vi "Insert Time Trace.vi"(4 "Anlaysis Info Cluster":T1={"Colour"=0, "Inst type"=enum."Pitot-static tube", "Inst name"="Manometer voltage", "Symbol"="U", "Code name"="", "Extra Info"="U", "Inst Array"=enum."PWA", "U"=0.0, "u^2"=0.0, "u^3"=0.0, "u^4"=0.0, "Skew_u"=0.0, "Kurt_u"=0.0, "Sd Error in Mean"=0.0, "% u'/U"=0.0, "X"=0.0, "Y"=0.0, "Z"=0.0, "Timescale integral Estimate"=0.0, "Sd Error in Variance"=0.0, "Calib File"=path "", "Calib Constants"=[], "Output Position"=FALSE, "Stats"=enum."None", "Av Sampling Rate"=0.0, "Av No of Samples"=0.0, "Total Meas Time (s)"=0.0, "OrigChName"="", "Max value"=0.0, "Min value"=0.0, "Req Sample Rate Hz"=0.0, "Sync Delay Time (s)"=0.0, "Ch No"=0, "Device"="", "Use Latest Calib"=FALSE, "Port"="", "Metadata Ch Names"=[], "Metadata Ch Values"=[], "Label"="", "chState"=enum."Solo", "Point Drift"=0.0, "inputConfig"=""} {"Kurt_u" format="%_3g"; "u^4" format="%_3g"; "u^3" format="%_3g"; "Sd Error in Variance" format="%_3g"; "u^2" format="%_3g"; "Sd Error in Mean" format="%_3g"; "U" format="%_3g"; "Sync Delay Time (s)" format="%.4f"; "Total Meas Time (s)" format="%_5g"; "Skew_u" format="%_3g"; "% u'/U" format="%_3g"}, 5 "No of Samples":i32, 6 "Total No of Chs":i32, 7 "Sampling Rate (Hz)":dbl, 8 "Time Trace In":T5, 9 "Input Array":dbl[](array[numeric]), 10 "Index":i32, 11 "Sync Delay (s)":dbl) -> (0 "Time Trace Out":T5)   [LabVIEW 2022 SP3]
uses:
  Controls/Time_Trace_Cluster.ctl
  Controls/Inst_type.ctl
  Controls/Analysis_info_cluster.ctl
  Controls/Instrument_Array.ctl
  Controls/channelState.ctl
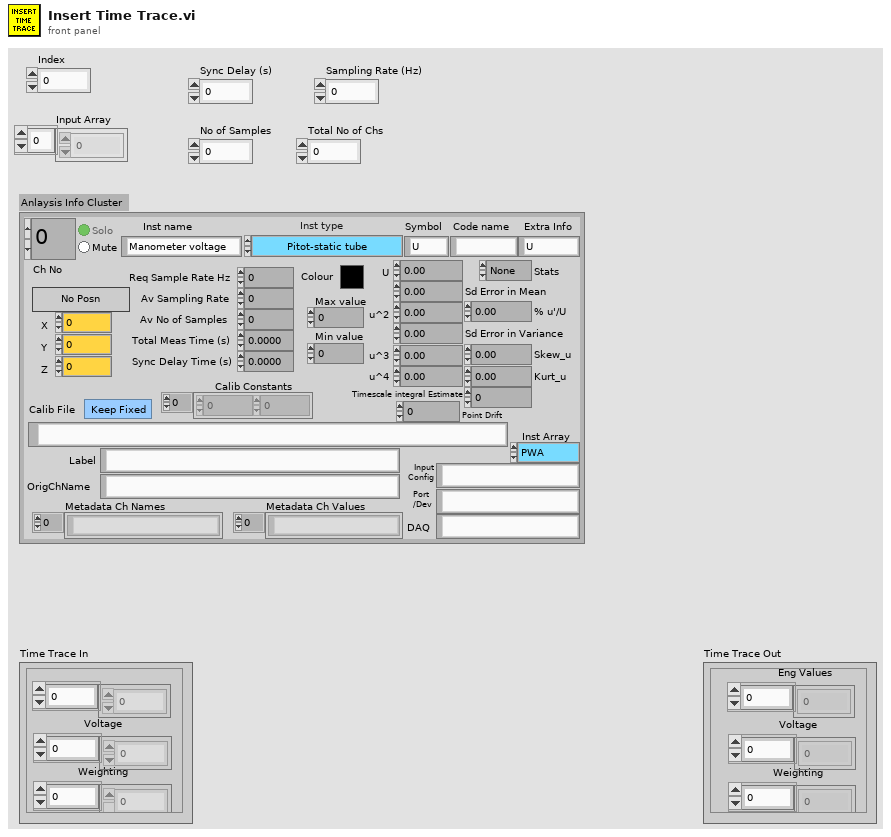
[diagram p1: front panel]
types:
  T1 = typedef "Analysis_info_cluster.ctl" = cluster{"Colour":u32, "Inst type":T2, "Inst name":string, "Symbol":string, "Code name":string, "Extra Info":string, "Inst Array":T3, "U":dbl, "u^2":dbl, "u^3":dbl, "u^4":dbl, "Skew_u":dbl, "Kurt_u":dbl, "Sd Error in Mean":dbl, "% u'/U":dbl, "X":dbl, "Y":dbl, "Z":dbl, "Timescale integral Estimate":dbl, "Sd Error in Variance":dbl, "Calib File":path, "Calib Constants":dbl[], "Output Position":bool, "Stats":enum16{"None", "Basic", "Full"}, "Av Sampling Rate":dbl, "Av No of Samples":dbl, "Total Meas Time (s)":dbl, "OrigChName":string, "Max value":dbl, "Min value":dbl, "Req Sample Rate Hz":dbl, "Sync Delay Time (s)":dbl, "Ch No":i16, "Device":string, "Use Latest Calib":bool, "Port":string, "Metadata Ch Names":string[], "Metadata Ch Values":string[], "Label":string, "chState":T4, "Point Drift":dbl, "inputConfig":string}
  T2 = typedef "Inst_type.ctl" = enum16{"Raw voltage", "Raw with zero offsetting", "Propeller anemometer", "Pressure Transducer", "Pitot-static tube", "Hot wire", "Cross wire 1", "Cross wire 2", "Generic Linear", "Generic Polynomial", "Generic BackPoly", "Fast FID", "Thermocouple", "Cold wire", "Pulsed Wire", "LDA Vel", "LDA Tran time", "LDA Arr time", "Microphone"}
  T3 = typedef "Instrument_Array.ctl" = enum16{"PWA", "LDA", "Analogue"}
  T4 = typedef "channelState.ctl" = enum32{"No Selection", "Solo", "Mute"}
  T5 = typedef "Time_Trace_Cluster.ctl" = cluster{"Weighting":dbl[], "Voltage":dbl[], "Eng Values":dbl[]}
  T6 = typedef "Data for Inst Type.ctl" = enum16{"Eng Values", "Voltage"}
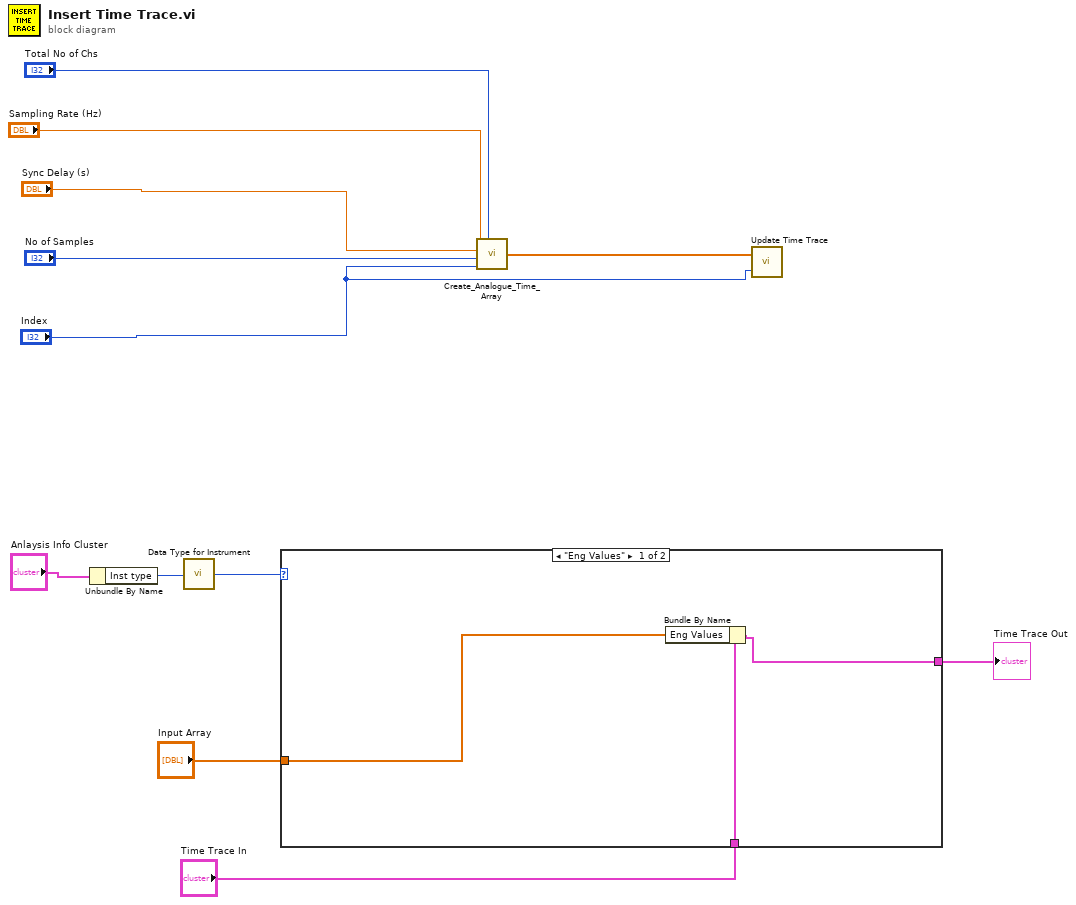
[diagram p0: block diagram]
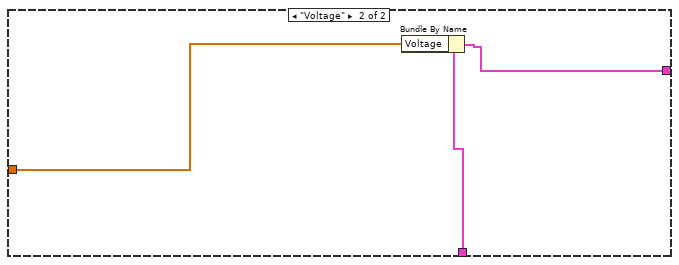
[diagram p2: hidden frame]
diagram:
  n1 = Unbundle By Name("Anlaysis Info Cluster") -> ("Inst type"=w4:T2)
  n2 = call "Data Type for Instrument.vi"("Inst type"=w4) -> ("Data for Inst Type"=w3:T6)
  n3 = case shown="\"Eng Values\"" w3 {
    tunnel: "Input Array" -> [w15 w18]
    tunnel: "Time Trace In" -> [w14 w17]
    tunnel: [w13 w16] -> w5
    frame "Eng Values" {
      n4 = Bundle By Name(cluster=w14, "Eng Values"=w15) -> (w13:T5)
    }
    frame "Voltage" {
      n5 = Bundle By Name(cluster=w17, "Voltage"=w18) -> (w16:T5)
    }
  }
  "Time Trace Out" <- w5
  n6 = call "Create_Analogue_Time_Array.vi"("Sampling Rate (Hz)"="Sampling Rate (Hz)", "Sync Delay (s)"="Sync Delay (s)", "No of Samples"="No of Samples", "Index"="Index", "Total No of Chs"="Total No of Chs") -> ("Times"=w2:dbl[])
  n7 = call "Update Time Trace.vi"("Channel Index"="Index", "Time (s)"=w2) -> ()  [unwired: 1 in]
